vi "Get Angle Limits.vi"(8 "error in (no error)":errorcluster, 11 "KUKA youBot arm motor in":refnum<class "NI_Robotics_KUKA youBot Arm Motor.lvclass">) -> (0 "error out":errorcluster, 1 "min angle (rad)":dbl, 2 "max angle (rad)":dbl, 3 "KUKA youBot arm motor out":refnum<class "NI_Robotics_KUKA youBot Arm Motor.lvclass">)   [LabVIEW 2017, in "NI_Robotics_KUKA youBot Host.lvlib" / "NI_Robotics_KUKA youBot Arm Motor.lvclass"]
uses:
  <vilib>/robotics/KUKA youBot/Motor/Arm Motor/NI_Robotics_KUKA youBot Arm Motor.lvclass
  <vilib>/robotics/KUKA youBot/Motor/Arm Motor/NI_Robotics_KUKA youBot Arm Motor.lvclass/NI_Robotics_KUKA youBot Arm Motor.ctl
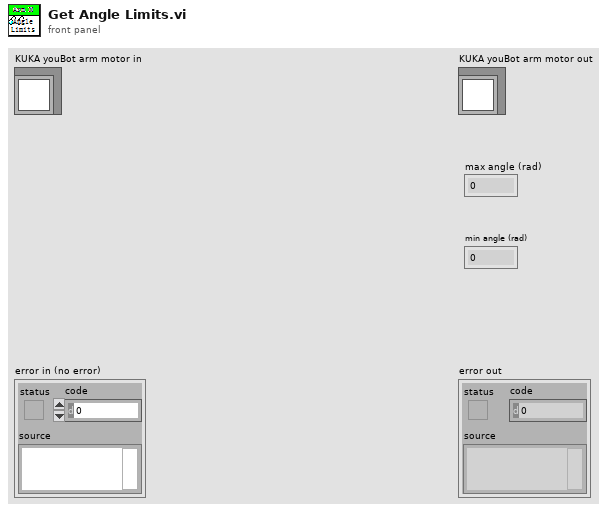
[diagram p1: front panel]
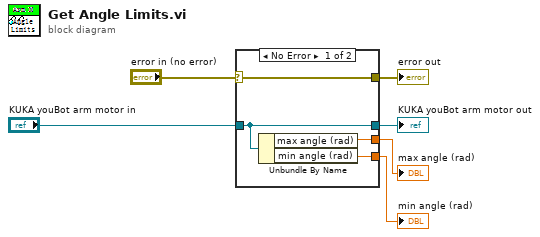
[diagram p0: block diagram]
diagram:
  n1 = case shown="No Error" "error in (no error)" {
    selector: "error in (no error)" -> [w10 w11]
    tunnel: [w10 w11] -> w5
    tunnel: [w9 w12] -> w3
    tunnel: "KUKA youBot arm motor in" -> [w9 w12]
    tunnel: [w8 _] -> w2
    tunnel: [w7 _] -> w1
    frame No Error {
      n2 = Unbundle By Name(w9) -> ("max angle (rad)"=w7:dbl, "min angle (rad)"=w8:dbl)
    }
    frame Error {
    }
  }
  "error out" <- w5
  "KUKA youBot arm motor out" <- w3
  "min angle (rad)" <- w2
  "max angle (rad)" <- w1
